vi "const trigger channel name.vi"() -> (3 "trigger channel":string)   [LabVIEW 2015, in "TDMS datalogger configuration.lvclass"]
uses:
  TDMS datalogger configuration.lvclass
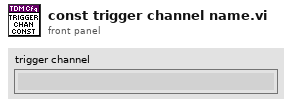
[diagram p1: front panel]
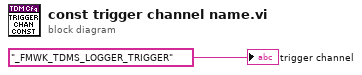
[diagram p0: block diagram]
diagram:
  "trigger channel" <- "_FMWK_TDMS_LOGGER_TRIGGER" ("enable channel")
